vi "Muti Area Capture.vi"() -> ()   [LabVIEW 2019]
doc: "This VI captures the region of the screen and displays it on the front panel continuously.\nCan be used to develop remote desktop applications."
uses:
  <vilib>/Utility/miscctls.llb/LVBoundsTypeDef.ctl
  System.Drawing
  <vilib>/Utility/inputDevices.llb/mouseAcquire.vi
  <vilib>/Utility/inputDevices.llb/closeMouse.vi
  <vilib>/wsapi/NI_WebServices.lvlib
panel:
  in  "Combo y offset":i32=150
  in  "Combo x offset":i32=-100
  out "Combo":picture
  in  "Combo  Height  (px)":i32=50
  in  "Combo Width (px)":i32=360
  in  "Bar y offset":i32=200
  in  "Bar x offset":i32=-70
  out "Bar":picture
  in  "Bar Height  (px)":i32=30
  in  "Bar Width (px)":i32=280
  in  "Space Height (px)":i32=60
  in  "Space Width (px)":i32=145
  out "Space":picture
  in  "stop":bool
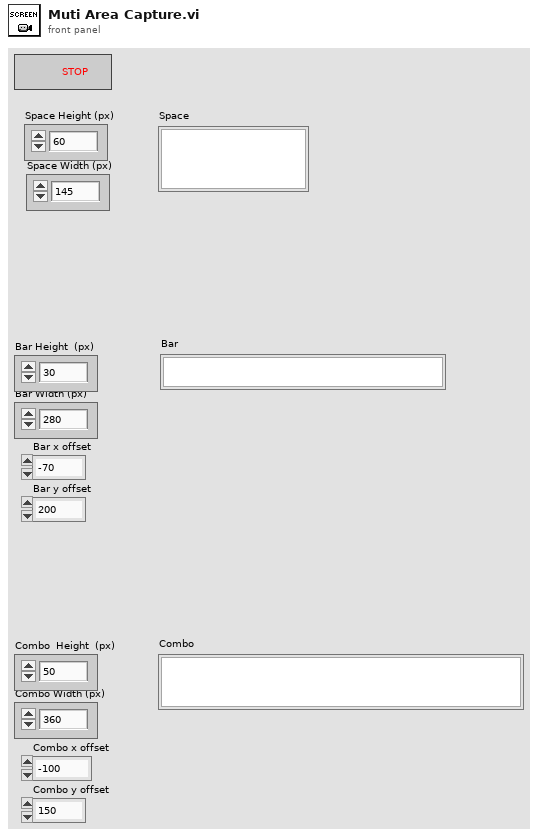
[diagram p1: front panel]
types:
  T1 = typedef "LVBoundsTypeDef.ctl" = cluster{"Width":u32, "Height":u32}
  T2 = cluster{"Horizontal":i32, "Vertical":i32, "Scrolling":i32}
  T3 = typedef "imagedata.ctl" = cluster{"image type":i32, "image depth":i32, "image":u8[], "mask":u8[], "colors":u32[], "Rectangle":cluster{"left":i16, "top":i16, "right":i16, "bottom":i16}}
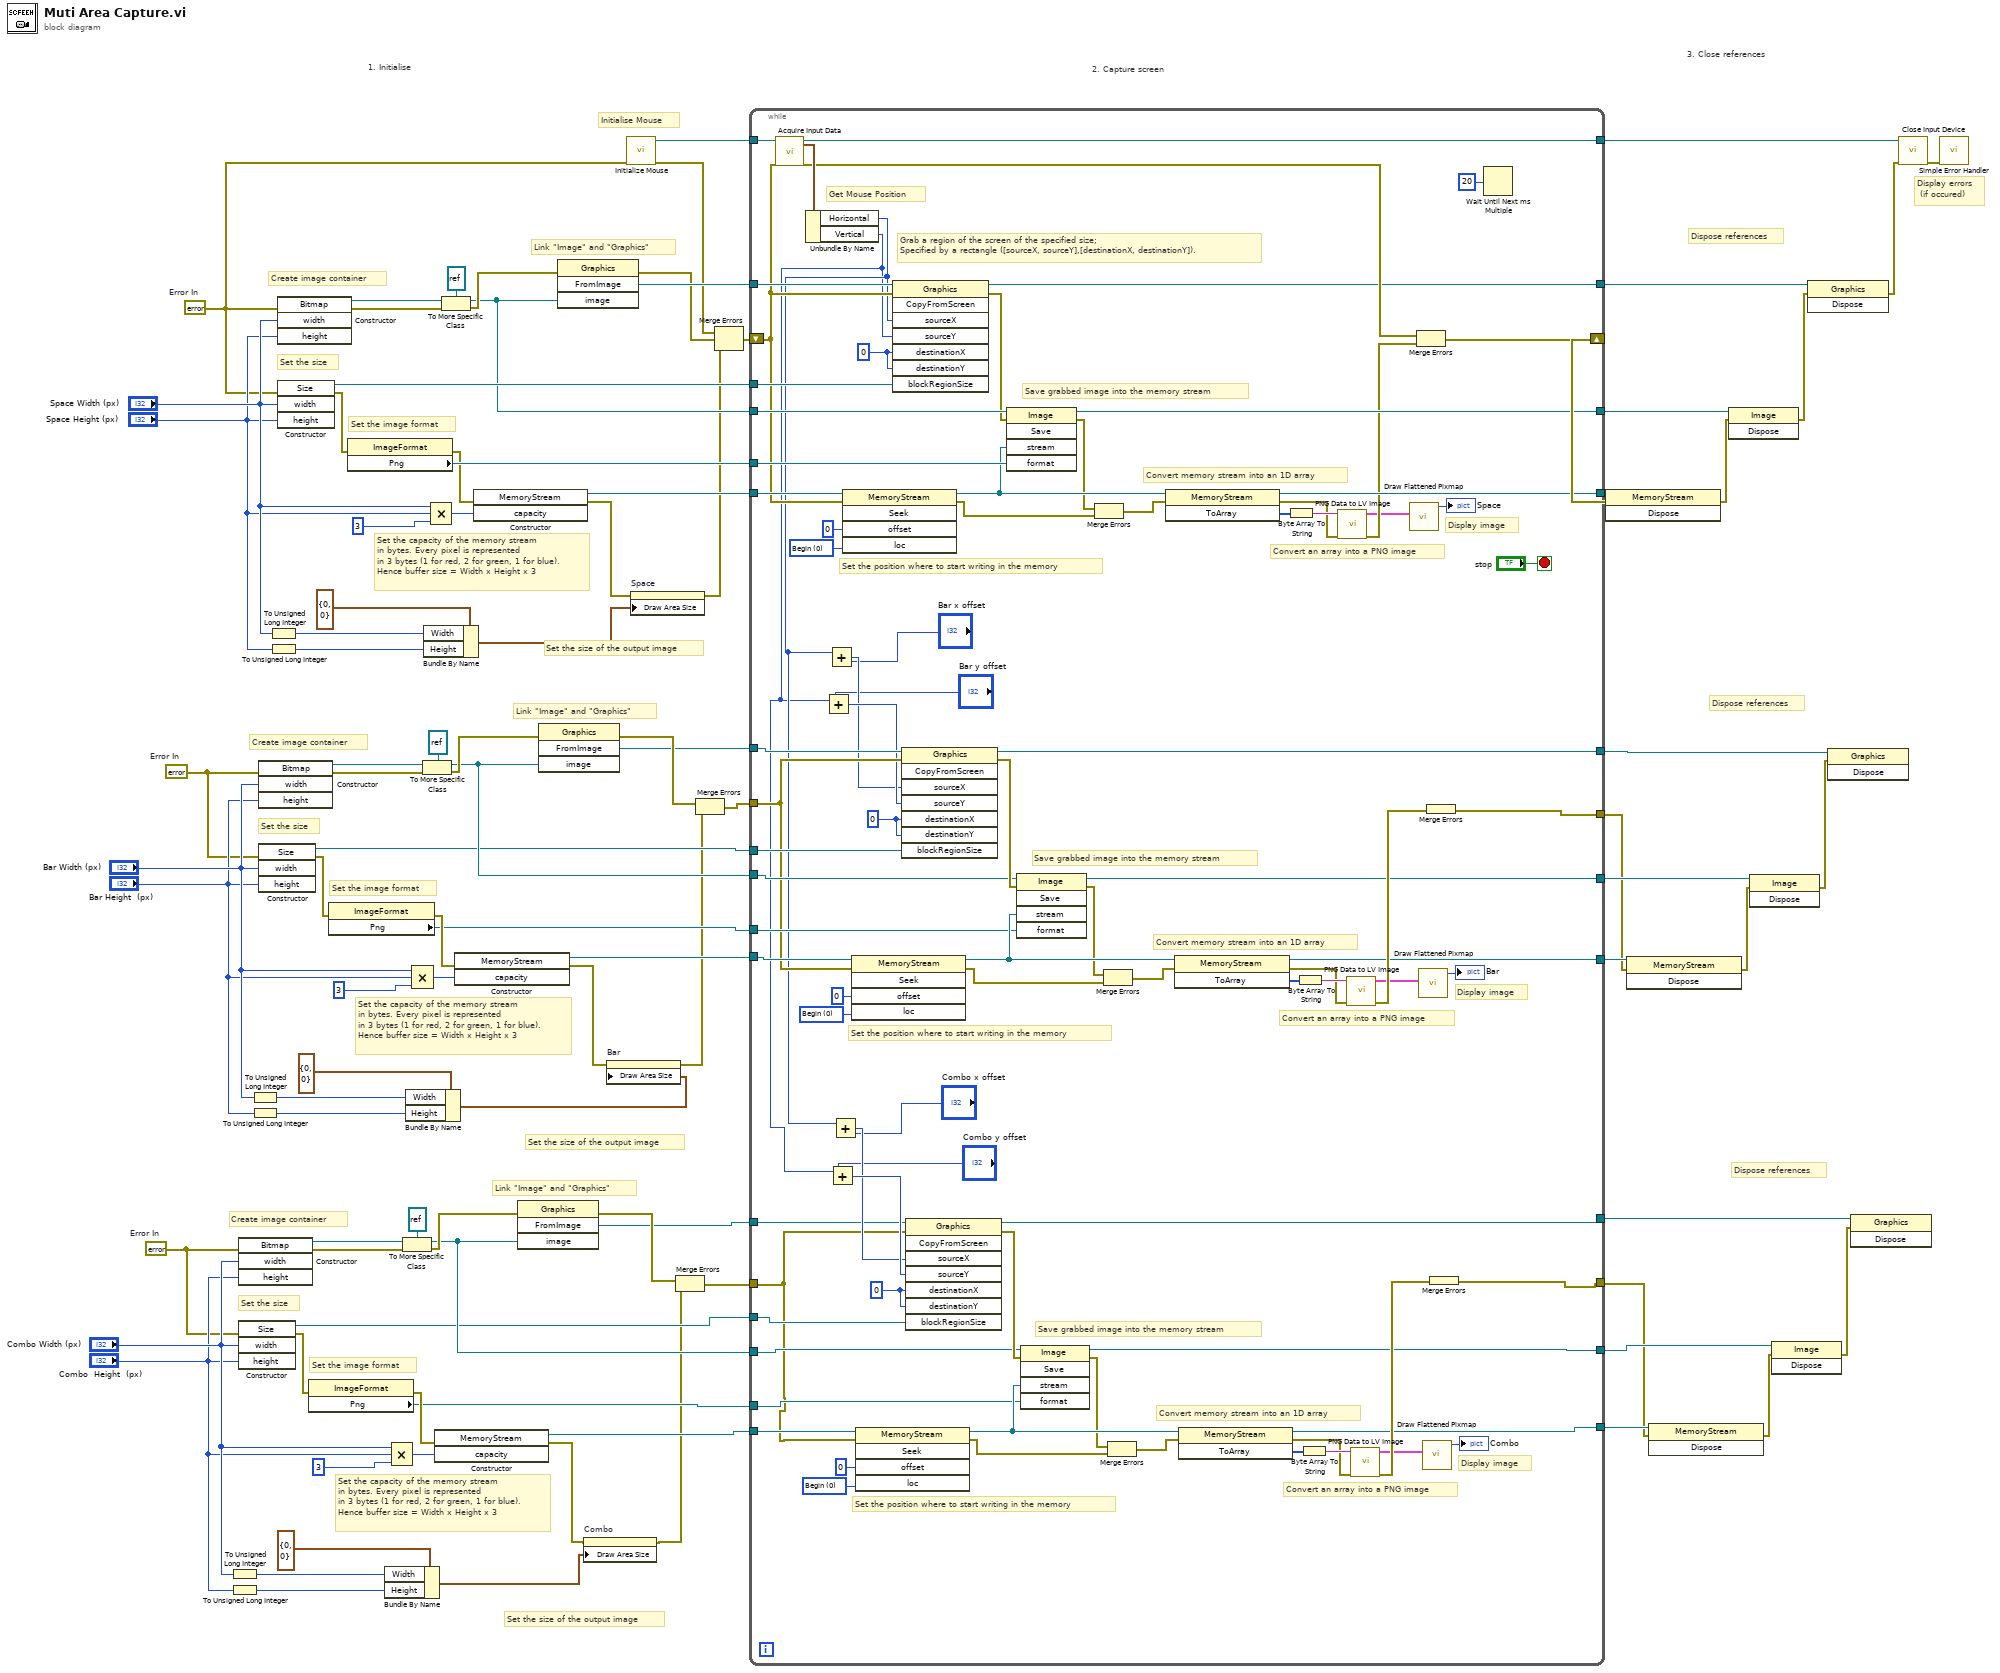
[diagram p0: block diagram]
diagram:
  w16 = errorcluster {"status"=FALSE, "code"=0, "source"=""}  # Error In
  w46 = errorcluster {"status"=FALSE, "code"=0, "source"=""}  # Error In
  w61 = errorcluster {"status"=FALSE, "code"=0, "source"=""}  # Error In
  # "Dispose references"
  # "Link \"Image\" and \"Graphics\""
  # "Set the size"
  # "Create image container"
  # "Set the image format"
  # "Set the size of the output image"
  # "Set the capacity of the memory stream\nin bytes. Every pixel is represented\nin 3 bytes (1 for red, 2 for green, 1 for blue).\nHence buffer size = Width x Height x 3"
  # "Dispose references"
  # "Link \"Image\" and \"Graphics\""
  # "Set the size"
  # "Create image container"
  # "Set the image format"
  # "Set the size of the output image"
  # "Set the capacity of the memory stream\nin bytes. Every pixel is represented\nin 3 bytes (1 for red, 2 for green, 1 for blue).\nHence buffer size = Width x Height x 3"
  # "Link \"Image\" and \"Graphics\""
  # "Set the size"
  # "Create image container"
  # "3. Close references"
  # "2. Capture screen"
  # "1. Initialise"
  # "Display errors\n (if occured)"
  # "Dispose references"
  # "Set the image format"
  # "Set the size of the output image"
  # "Set the capacity of the memory stream\nin bytes. Every pixel is represented\nin 3 bytes (1 for red, 2 for green, 1 for blue).\nHence buffer size = Width x Height x 3"
  # "Initialise Mouse"
  n1 = To Unsigned Long Integer(number="Combo Width (px)") -> (unsigned 32bit integer=w19:u32)
  n2 = To Unsigned Long Integer(number="Combo  Height  (px)") -> (unsigned 32bit integer=w17:u32)
  n3 = constructor class="Bitmap"(error in=w16, "width"="Combo Width (px)", "height"="Combo  Height  (px)") -> (reference out=w27:refnum<k24>, error out=w29:errorcluster)  [unwired: 2 in, 3 out]
  n4 = constructor class="Size"(error in=w16, "width"="Combo Width (px)", "height"="Combo  Height  (px)") -> (reference out=w12:refnum<k24>, error out=w23:errorcluster)  [unwired: 2 in, 3 out]
  n5 = To Unsigned Long Integer(number="Bar Width (px)") -> (unsigned 32bit integer=w49:u32)
  n6 = To Unsigned Long Integer(number="Bar Height  (px)") -> (unsigned 32bit integer=w47:u32)
  n7 = constructor class="Bitmap"(error in=w46, "width"="Bar Width (px)", "height"="Bar Height  (px)") -> (reference out=w57:refnum<k24>, error out=w59:errorcluster)  [unwired: 2 in, 3 out]
  n8 = constructor class="Size"(error in=w46, "width"="Bar Width (px)", "height"="Bar Height  (px)") -> (reference out=w42:refnum<k24>, error out=w53:errorcluster)  [unwired: 2 in, 3 out]
  n9 = To Unsigned Long Integer(number="Space Width (px)") -> (unsigned 32bit integer=w69:u32)
  n10 = To Unsigned Long Integer(number="Space Height (px)") -> (unsigned 32bit integer=w67:u32)
  n11 = constructor class="Bitmap"(error in=w61, "width"="Space Width (px)", "height"="Space Height (px)") -> (reference out=w89:refnum<k24>, error out=w92:errorcluster)  [unwired: 2 in, 3 out]
  n12 = constructor class="Size"(error in=w61, "width"="Space Width (px)", "height"="Space Height (px)") -> (reference out=w87:refnum<k24>, error out=w78:errorcluster)  [unwired: 2 in, 3 out]
  n13 = property class="ImageFormat"(error in=w23) -> (error out=w22:errorcluster, "Png"=w14:refnum<k24>)  [unwired: 1 in, 1 out]
  n14 = property class="ImageFormat"(error in=w53) -> (error out=w52:errorcluster, "Png"=w44:refnum<k24>)  [unwired: 1 in, 1 out]
  n15 = property class="ImageFormat"(error in=w78) -> (error out=w77:errorcluster, "Png"=w86:refnum<k24>)  [unwired: 1 in, 1 out]
  n16 = Bundle By Name(cluster=T1 {"Width"=0, "Height"=0} ("Draw Area Size"), "Width"=w19, "Height"=w17) -> (w3:T1)
  n17 = Compound Arithmetic op=MULTIPLY("Combo Width (px)", "Combo  Height  (px)", 3 ("value")) -> (w25:i32)
  n18 = To More Specific Class(target class=refnum<k24> refnum, reference=w27, error in=w29) -> (specific class reference=w13:refnum<k24>, error out=w30:errorcluster)
  n19 = Bundle By Name(cluster=T1 {"Width"=0, "Height"=0} ("Draw Area Size"), "Width"=w49, "Height"=w47) -> (w31:T1)
  n20 = Compound Arithmetic op=MULTIPLY("Bar Width (px)", "Bar Height  (px)", 3 ("value")) -> (w55:i32)
  n21 = To More Specific Class(target class=refnum<k24> refnum, reference=w57, error in=w59) -> (specific class reference=w43:refnum<k24>, error out=w60:errorcluster)
  n22 = Bundle By Name(cluster=T1 {"Width"=0, "Height"=0} ("Draw Area Size"), "Width"=w69, "Height"=w67) -> (w73:T1)
  n23 = Compound Arithmetic op=MULTIPLY("Space Width (px)", "Space Height (px)", 3 ("value")) -> (w81:i32)
  n24 = constructor class="MemoryStream"(error in=w22, "capacity"=w25) -> (reference out=w15:refnum<k24>, error out=w2:errorcluster)  [unwired: 2 in, 2 out]
  n25 = To More Specific Class(target class=refnum<k24> refnum, reference=w89, error in=w92) -> (specific class reference=w80:refnum<k24>, error out=w93:errorcluster)
  n26 = constructor class="MemoryStream"(error in=w52, "capacity"=w55) -> (reference out=w45:refnum<k24>, error out=w32:errorcluster)  [unwired: 2 in, 2 out]
  n27 = constructor class="MemoryStream"(error in=w77, "capacity"=w81) -> (reference out=w83:refnum<k24>, error out=w72:errorcluster)  [unwired: 2 in, 2 out]
  n28 = invoke class="Graphics" method="FromImage"(error in=w30, "image"=w13) -> (error out=w21:errorcluster, "FromImage"=w11:refnum<k24>)  [unwired: 2 in, 2 out]
  n29 = invoke class="Graphics" method="FromImage"(error in=w60, "image"=w43) -> (error out=w51:errorcluster, "FromImage"=w41:refnum<k24>)  [unwired: 2 in, 2 out]
  n30 = invoke class="Graphics" method="FromImage"(error in=w93, "image"=w80) -> (error out=w76:errorcluster, "FromImage"=w90:refnum<k24>)  [unwired: 2 in, 2 out]
  n31 = property on="Combo" class="Pict"(error in=w2, "Draw Area Size"=w3) -> (error out=w1:errorcluster)  [unwired: 1 in, 1 out]
  n32 = property on="Bar" class="Pict"(error in=w32, "Draw Area Size"=w31) -> (error out=w33:errorcluster)  [unwired: 1 in, 1 out]
  n33 = call <vilib>:"Initialize Mouse.vi"("error in (no error)"=w61) -> ("error out"=w74:errorcluster, "device ID"=w95:refnum<k1>)  [unwired: 9 in]
  n34 = property on="Space" class="Pict"(error in=w72, "Draw Area Size"=w73) -> (error out=w71:errorcluster)  [unwired: 1 in, 1 out]
  n35 = Merge Errors(w21, w1) -> (w10:errorcluster)
  n36 = Merge Errors(w51, w33) -> (w40:errorcluster)
  n37 = Merge Errors(w74, w76, w71) -> (w75:errorcluster)
  n38 = while {
    tunnel: w95 -> [w183]
    tunnel: [w181] -> w94
    tunnel: w90 -> [w180]
    tunnel: [w177] -> w88
    tunnel: w87 -> [w176]
    tunnel: w86 -> [w175]
    tunnel: [w174] -> w85
    tunnel: w83 -> [w173]
    tunnel: w80 -> [w166]
    shift-right: [w157] -> w66
    shift-left: w75 -> [w160]
    tunnel: [w156] -> w65
    tunnel: w45 -> [w139]
    tunnel: w44 -> [w138]
    tunnel: w43 -> [w137]
    tunnel: w42 -> [w136]
    tunnel: w41 -> [w135]
    tunnel: w40 -> [w134]
    tunnel: [w133] -> w37
    tunnel: [w132] -> w36
    tunnel: [w131] -> w35
    tunnel: [w130] -> w34
    tunnel: w15 -> [w107]
    tunnel: w14 -> [w106]
    tunnel: w13 -> [w105]
    tunnel: w12 -> [w104]
    tunnel: w11 -> [w103]
    tunnel: w10 -> [w102]
    tunnel: [w99] -> w7
    tunnel: [w98] -> w6
    tunnel: [w97] -> w5
    tunnel: [w96] -> w4
    stop <- "stop" stop-if-true
    w119 = 0 ("destinationX")
    w122 = 0 items=["Begin", "Current", "End"] ("loc")
    w147 = 0 ("destinationX")
    w150 = 0 items=["Begin", "Current", "End"] ("loc")
    w167 = 0 ("destinationX")
    w171 = 0 items=["Begin", "Current", "End"] ("loc")
    # "Display image"
    # "Convert an array into a PNG image"
    # "Set the position where to start writing in the memory"
    # "Convert memory stream into an 1D array"
    # "Save grabbed image into the memory stream"
    # "Display image"
    # "Convert an array into a PNG image"
    # "Set the position where to start writing in the memory"
    # "Convert memory stream into an 1D array"
    # "Save grabbed image into the memory stream"
    # "Display image"
    # "Convert an array into a PNG image"
    # "Set the position where to start writing in the memory"
    # "Convert memory stream into an 1D array"
    # "Save grabbed image into the memory stream"
    # "Grab a region of the screen of the specified size;\nSpecified by a rectangle ([sourceX, sourceY],[destinationX, destinationY])."
    # "Get Mouse Position"
    n39 = call-poly <vilib>:"Acquire Input Data.vi"("device ID"=w183, "error in (no error)"=w160) -> ("device ID"=w181:refnum<k1>, "axis info"=w182:T2, "error out"=w159:errorcluster)  [unwired: 14 in, 1 out]
    n40 = Unbundle By Name(w182) -> ("Horizontal"=w101:i32, "Vertical"=w100:i32)
    n41 = Add(x=w100, y="Bar y offset") -> (x+y=w129:i32)
    n42 = Add(x=w101, y="Bar x offset") -> (x+y=w128:i32)
    n43 = Add(x=w100, y="Combo y offset") -> (x+y=w111:i32)
    n44 = Add(x=w101, y="Combo x offset") -> (x+y=w110:i32)
    n45 = invoke class="MemoryStream" method="Seek"(reference=w173, error in=w160, "offset"=i64 0, "loc"=w171) -> (reference out=w168:refnum<k24>, error out=w163:errorcluster)  [unwired: 1 in, 3 out]
    n46 = invoke class="MemoryStream" method="Seek"(reference=w139, error in=w134, "offset"=i64 0, "loc"=w150) -> (reference out=w148:refnum<k24>, error out=w144:errorcluster)  [unwired: 1 in, 3 out]
    n47 = invoke class="MemoryStream" method="Seek"(reference=w107, error in=w102, "offset"=i64 0, "loc"=w122) -> (reference out=w120:refnum<k24>, error out=w116:errorcluster)  [unwired: 1 in, 3 out]
    n48 = invoke class="Graphics" method="CopyFromScreen"(reference=w180, error in=w160, "sourceX"=w101, "sourceY"=w100, "destinationX"=w167, "destinationY"=w167, "blockRegionSize"=w176) -> (reference out=w156:refnum<k24>, error out=w161:errorcluster)  [unwired: 1 in, 6 out]
    n49 = invoke class="Graphics" method="CopyFromScreen"(reference=w135, error in=w134, "sourceX"=w128, "sourceY"=w129, "destinationX"=w147, "destinationY"=w147, "blockRegionSize"=w136) -> (reference out=w132:refnum<k24>, error out=w142:errorcluster)  [unwired: 1 in, 6 out]
    n50 = invoke class="Graphics" method="CopyFromScreen"(reference=w103, error in=w102, "sourceX"=w110, "sourceY"=w111, "destinationX"=w119, "destinationY"=w119, "blockRegionSize"=w104) -> (reference out=w96:refnum<k24>, error out=w114:errorcluster)  [unwired: 1 in, 6 out]
    n51 = invoke class="Image" method="Save"(reference=w166, error in=w161, "stream"=w168, "format"=w175) -> (reference out=w174:refnum<k24>, error out=w164:errorcluster)  [unwired: 1 in, 3 out]
    n52 = invoke class="Image" method="Save"(reference=w137, error in=w142, "stream"=w148, "format"=w138) -> (reference out=w133:refnum<k24>, error out=w145:errorcluster)  [unwired: 1 in, 3 out]
    n53 = invoke class="Image" method="Save"(reference=w105, error in=w114, "stream"=w120, "format"=w106) -> (reference out=w98:refnum<k24>, error out=w117:errorcluster)  [unwired: 1 in, 3 out]
    n54 = Merge Errors(w164, w163) -> (w162:errorcluster)
    n55 = Merge Errors(w145, w144) -> (w143:errorcluster)
    n56 = Merge Errors(w117, w116) -> (w115:errorcluster)
    n57 = invoke class="MemoryStream" method="ToArray"(reference=w168, error in=w162) -> (reference out=w177:refnum<k24>, error out=w165:errorcluster, "ToArray"=w179:u8[])  [unwired: 1 in]
    n58 = invoke class="MemoryStream" method="ToArray"(reference=w148, error in=w143) -> (reference out=w131:refnum<k24>, error out=w146:errorcluster, "ToArray"=w153:u8[])  [unwired: 1 in]
    n59 = invoke class="MemoryStream" method="ToArray"(reference=w120, error in=w115) -> (reference out=w99:refnum<k24>, error out=w118:errorcluster, "ToArray"=w125:u8[])  [unwired: 1 in]
    n60 = Byte Array To String(unsigned byte array=w179) -> (string=w178:string)
    n61 = Byte Array To String(unsigned byte array=w153) -> (string=w152:string)
    n62 = Byte Array To String(unsigned byte array=w125) -> (string=w124:string)
    n63 = call <vilib>:"PNG Data to LV Image.vi"("error in (no error)"=w165, "png data"=w178) -> ("error out"=w158:errorcluster, "image data"=w155:T3)  [unwired: 8 in]
    n64 = call <vilib>:"PNG Data to LV Image.vi"("error in (no error)"=w146, "png data"=w152) -> ("error out"=w141:errorcluster, "image data"=w140:T3)  [unwired: 8 in]
    n65 = call <vilib>:"PNG Data to LV Image.vi"("error in (no error)"=w118, "png data"=w124) -> ("error out"=w113:errorcluster, "image data"=w112:T3)  [unwired: 8 in]
    n66 = call <vilib>:"Draw Flattened Pixmap.vi"("image data"=w155) -> ("new picture"=→"Space":picture)  [unwired: 8 in]
    n67 = Merge Errors(w159, w158) -> (w157:errorcluster)
    n68 = call <vilib>:"Draw Flattened Pixmap.vi"("image data"=w140) -> ("new picture"=→"Bar":picture)  [unwired: 8 in]
    n69 = call <vilib>:"Draw Flattened Pixmap.vi"("image data"=w112) -> ("new picture"=→"Combo":picture)  [unwired: 8 in]
    n70 = Merge Errors(w141) -> (w130:errorcluster)
    n71 = Merge Errors(w113) -> (w97:errorcluster)
    n72 = Wait Until Next ms Multiple(millisecond multiple=u32 20) -> ()  [unwired: 1 out]
  }
  n73 = invoke class="MemoryStream" method="Dispose"(reference=w88, error in=w66) -> (error out=w84:errorcluster)  [unwired: 1 in, 2 out]
  n74 = invoke class="MemoryStream" method="Dispose"(reference=w35, error in=w34) -> (error out=w39:errorcluster)  [unwired: 1 in, 2 out]
  n75 = invoke class="MemoryStream" method="Dispose"(reference=w7, error in=w5) -> (error out=w9:errorcluster)  [unwired: 1 in, 2 out]
  n76 = invoke class="Image" method="Dispose"(reference=w85, error in=w84) -> (error out=w64:errorcluster)  [unwired: 1 in, 2 out]
  n77 = invoke class="Image" method="Dispose"(reference=w37, error in=w39) -> (error out=w38:errorcluster)  [unwired: 1 in, 2 out]
  n78 = invoke class="Image" method="Dispose"(reference=w6, error in=w9) -> (error out=w8:errorcluster)  [unwired: 1 in, 2 out]
  n79 = invoke class="Graphics" method="Dispose"(reference=w65, error in=w64) -> (error out=w63:errorcluster)  [unwired: 1 in, 2 out]
  n80 = invoke class="Graphics" method="Dispose"(reference=w36, error in=w38) -> ()  [unwired: 1 in, 3 out]
  n81 = invoke class="Graphics" method="Dispose"(reference=w4, error in=w8) -> ()  [unwired: 1 in, 3 out]
  n82 = call-poly <vilib>:"Close Input Device.vi"("error in (no error)"=w63, "device ID"=w94) -> ("error out"=w62:errorcluster)  [unwired: 8 in]
  n83 = call <vilib>:"Simple Error Handler.vi"("error in (no error)"=w62) -> ()  [unwired: 4 in, 5 out]
